vi "merge configuration with system.vi"(8 "error in":errorcluster, 11 "Scan Engine configuration in":refnum<class "Scan Engine configuration.lvclass">) -> (0 "error out":errorcluster, 3 "Scan Engine configuration out":refnum<class "Scan Engine configuration.lvclass">)   [LabVIEW 2013, in "Scan Engine runtime.lvclass"]
uses:
  Scan Engine runtime.lvclass
  configuration/Scan Engine configuration.lvclass
  <vilib>/NI/Tag Bus Module Framework/channel/channel classification.ctl
  <vilib>/NI/Tag Bus Module Framework/channel/TBM channel.lvclass/TBM channel.ctl
  <vilib>/NI/Tag Bus/tag/tag descriptor.lvclass/tag descriptor.ctl
  <vilib>/NI/Tag Bus/tag/write data type.vi
  <vilib>/NI/Tag Bus Module Framework/channel/Write channel classification.vi
  <vilib>/NI/Tag Bus Module Framework/channel/Read channel classification.vi
  <vilib>/NI/Tag Bus/tag/read data type.vi
  <vilib>/NI/Tag Bus Module Framework/channel/TBM channel.lvclass
  <vilib>/NI/Configuration Framework/NISE_CEF_TreeControl.lvlib
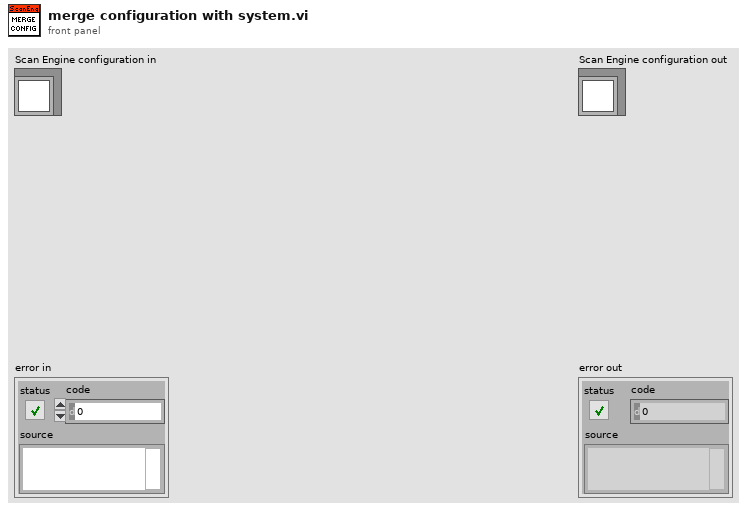
[diagram p1: front panel]
types:
  T1 = typedef "Scan Engine runtime.lvclass/system variable.ctl" = cluster{"reference":refnum<k21>, "data type":T2, "Writable":bool}
  T2 = typedef "tag bus.lvlib/tag descriptor.lvclass/Data Type.ctl" = enum16{"Double", "Single", "I64", "I32", "I16", "I8", "U64", "U32", "U16", "U8", "Boolean", "String", "Array of Double", "Array of Single", "Array of I64", "Array of I32", "Array of I16", "Array of I8", "Array of U64", "Array of U32", "Array of U16", "Array of U8", "Array of Boolean", "Array of String"}
  T3 = typedef "TBM channel.lvclass/channel classification.ctl" = enum16{"input data", "output data", "processing parameter", "processing result"}
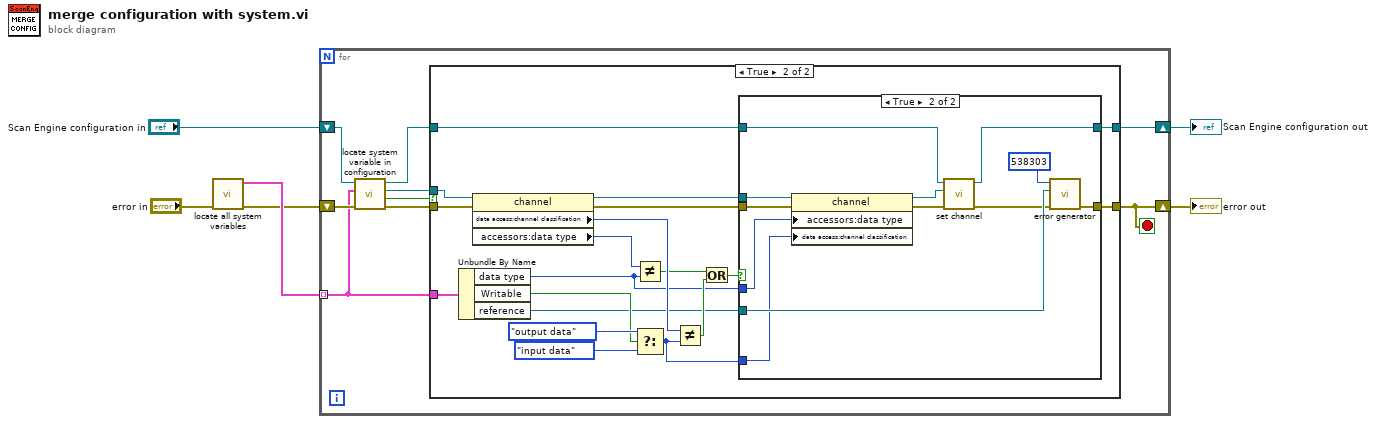
[diagram p0: block diagram]
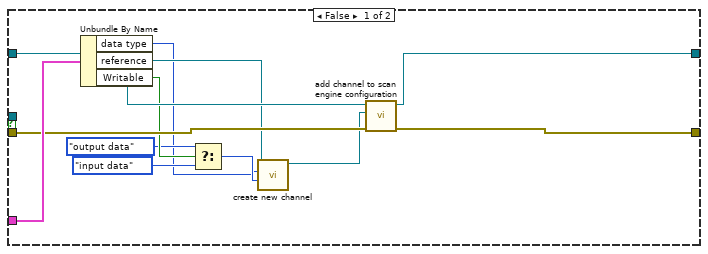
[diagram p2: hidden frame]
diagram:
  n1 = call "locate all system variables.vi"("error in"="error in") -> ("error out"=w1:errorcluster, "system variables"=w3:T1[])  [unwired: 9 in]
  n2 = for {
    shift-right: [w8] -> w5
    shift-left: "Scan Engine configuration in" -> [w15]
    shift-right: [w7] -> w4
    shift-left: w1 -> [w14]
    tunnel: w3 -> [w9] mode=indexing
    stop <- w7 stop-if-true
    n3 = call "locate system variable in configuration.vi"("error in"=w14, "raw variable data"=w9, "Scan Engine configuration in"=w15) -> ("error out"=w12:errorcluster, "found?"=w13:bool, "channel"=w10:refnum<class "TBM channel.lvclass">, "Scan Engine configuration out"=w11:refnum<class "Scan Engine configuration.lvclass">)  [unwired: 5 in]
    n4 = case shown="True" w13 {
      tunnel: w12 -> [w25 w42]
      tunnel: w11 -> [w27 w34]
      tunnel: w10 -> [_ w41]
      tunnel: w9 -> [w26 w46]
      tunnel: [w21 w32] -> w7
      tunnel: [w20 w35] -> w8
      frame False {
        n5 = Unbundle By Name(w26) -> ("data type"=w17:T2, "reference"=w18:refnum<k21>, "Writable"=w24:bool)
        n6 = Select(t=channel_classification."output data" ("channel classification"), s=w24, f=channel_classification."input data" ("channel classification")) -> (s? t:f=w19:T3)
        n7 = call <vilib>:"create new channel.vi"("channel classification"=w19, "data type"=w17, "channel name"=w18) -> ("channel"=w16:refnum<class "TBM channel.lvclass">)  [unwired: 8 in]
        n8 = call "add channel to scan engine configuration.vi"("error in"=w25, "channel"=w16, "Scan Engine configuration in"=w27) -> ("error out"=w21:errorcluster, "Scan Engine configuration out"=w20:refnum<class "Scan Engine configuration.lvclass">)  [unwired: 7 in]
      }
      frame True {
        n9 = Unbundle By Name(w46) -> ("data type"=w28:T2, "Writable"=w43:bool, "reference"=w31:refnum<k21>)
        n10 = property class="channel"(reference=w41, error in=w42) -> (reference out=w30:refnum<class "TBM channel.lvclass">, error out=w33:errorcluster, "data access:channel classification"=w39:T3, "accessors:data type"=w40:T2)
        n11 = Not Equal?(x=w40, y=w28) -> (x != y?=w37:bool)
        n12 = Select(t=channel_classification."output data" ("channel classification"), s=w43, f=channel_classification."input data" ("channel classification")) -> (s? t:f=w29:T3)
        n13 = Not Equal?(x=w39, y=w29) -> (x != y?=w38:bool)
        n14 = Or(x=w37, y=w38) -> (x .or. y?=w36:bool)
        n15 = case shown="True" w36 {
          tunnel: [w48 w50] -> w35
          tunnel: w34 -> [w48 w49]
          tunnel: w33 -> [w47 w56]
          tunnel: [w47 w59] -> w32
          tunnel: w31 -> [_ w58]
          tunnel: w30 -> [_ w57]
          tunnel: w29 -> [_ w54]
          tunnel: w28 -> [_ w55]
          frame False {
          }
          frame True {
            n16 = property class="channel"(reference=w57, error in=w56, "accessors:data type"=w55, "data access:channel classification"=w54) -> (reference out=w53:refnum<class "TBM channel.lvclass">, error out=w52:errorcluster)
            n17 = call "set channel.vi"("error in"=w52, "channel"=w53, "Scan Engine configuration in"=w49) -> ("error out"=w51:errorcluster, "Scan Engine configuration out"=w50:refnum<class "Scan Engine configuration.lvclass">)  [unwired: 7 in]
            n18 = call <vilib>:"error generator.vi"("error in"=w51, "append error message"=w58, "error code (0)"=538303) -> ("error out"=w59:errorcluster)  [unwired: 6 in]
          }
        }
      }
    }
  }
  "Scan Engine configuration out" <- w5
  "error out" <- w4
